vi "Actor Core.vi"(8 "error in":errorcluster, 11 "SongPlayerActor in":refnum<class "SongPlayerActor.lvclass">) -> (0 "error out":errorcluster, 3 "Actor out":refnum<class "Actor.lvclass">)   [LabVIEW 2015, in "SongPlayerActor.lvlib" / "SongPlayerActor.lvclass"]
doc: "(<B>Filename</B>: Actor Framework.lvlib:Actor.lvclass:Actor Core.vi)\n\nReceives messages to the actor, reacts to them, and initiates any error handling that may shut the actor down.\n\nDescendant classes may override this VI to append parallel tasks for the actor to complete while it handles messages. Overrides use the Call Parent Method node."
uses:
  SongPlayerActor.lvclass
  <vilib>/ActorFramework/Actor/Actor.lvclass
  file/MusicElement/Song/Song Duration.ctl
  file/MusicElement/Song/Song.lvclass
  SongPlayerActor.lvclass/SongPlayerActor.ctl
  <vilib>/ActorFramework/Actor/Actor.lvclass/Actor.ctl
  <vilib>/ActorFramework/Message Enqueuer/Message Enqueuer.lvclass/Message Enqueuer.ctl
  file/MusicElement/Song/Song.lvclass/Song.ctl
  file/MusicElement/MusicElement.lvclass/MusicElement.ctl
  file/MusicElement/Read Name.vi
  file/MusicElement/Song/Read Artist.vi
  file/MusicElement/Song/Read Album.vi
  <vilib>/ActorFramework/Message Enqueuer/Init from Existing Queue.vi
  <vilib>/ActorFramework/Message Enqueuer/Enqueue.vi
  <vilib>/ActorFramework/Message Priority Queue/Priority Enqueue.vi
  <vilib>/ActorFramework/Message Enqueuer/Message Enqueuer.lvclass
  <vilib>/ActorFramework/Stop Msg/Stop Msg.lvclass
  SongQueueActor/SongQueueActor Messages/Dequeue Next Song Msg/Dequeue Next Song Msg.lvclass
  SongQueueActor/SongQueueActor Messages/Play Previous Song Msg/Play Previous Song Msg.lvclass
panel:
  out "Main UI":enum32{"Main", "Debug"}(tab)
  out "Time Remaining (s)":T1 format="%<%M:%S>T"
  in  "Song Progress (%)":dbl(slide) scale=0.0..1.0
  in  "Paused?":bool
  in  "Previous Song":bool
  in  "Next Song":bool
  out "Artist":string
  out "Album":string
  out "Song Name":string
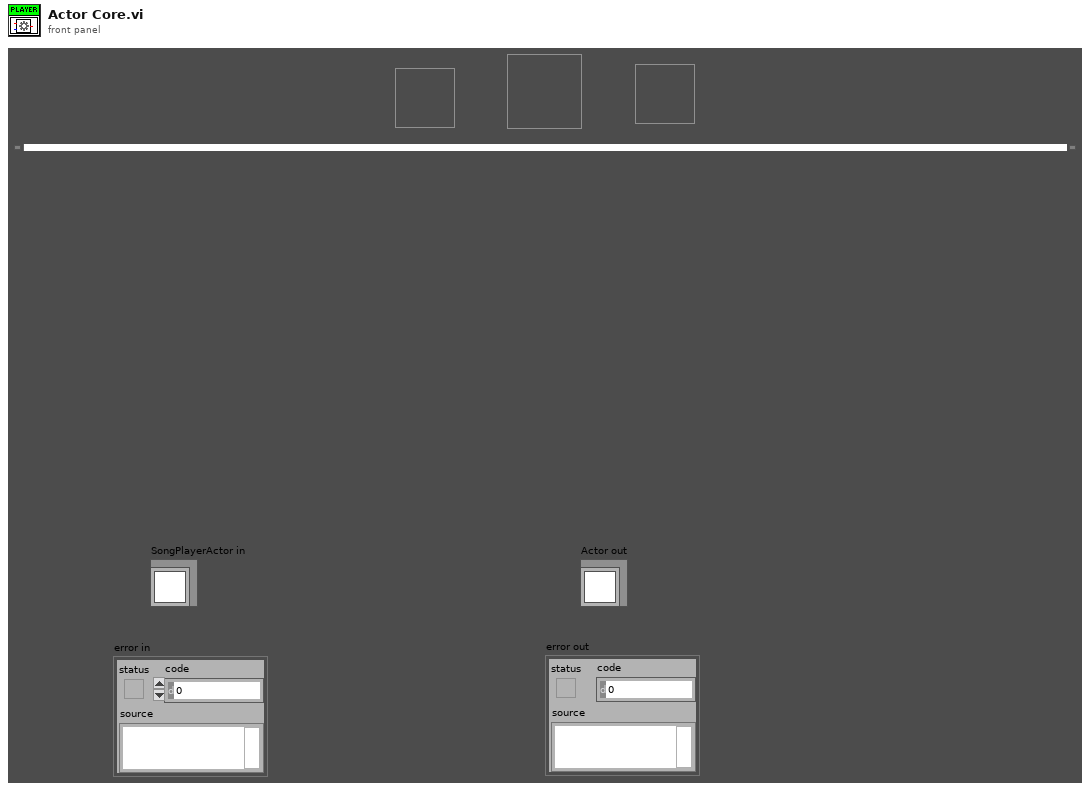
[diagram p1: front panel]
types:
  T1 = typedef "Song.lvclass/Song Duration.ctl" = timestamp
  T2 = enum8{"Enabled", "Disabled", "Disabled and Grayed Out"}
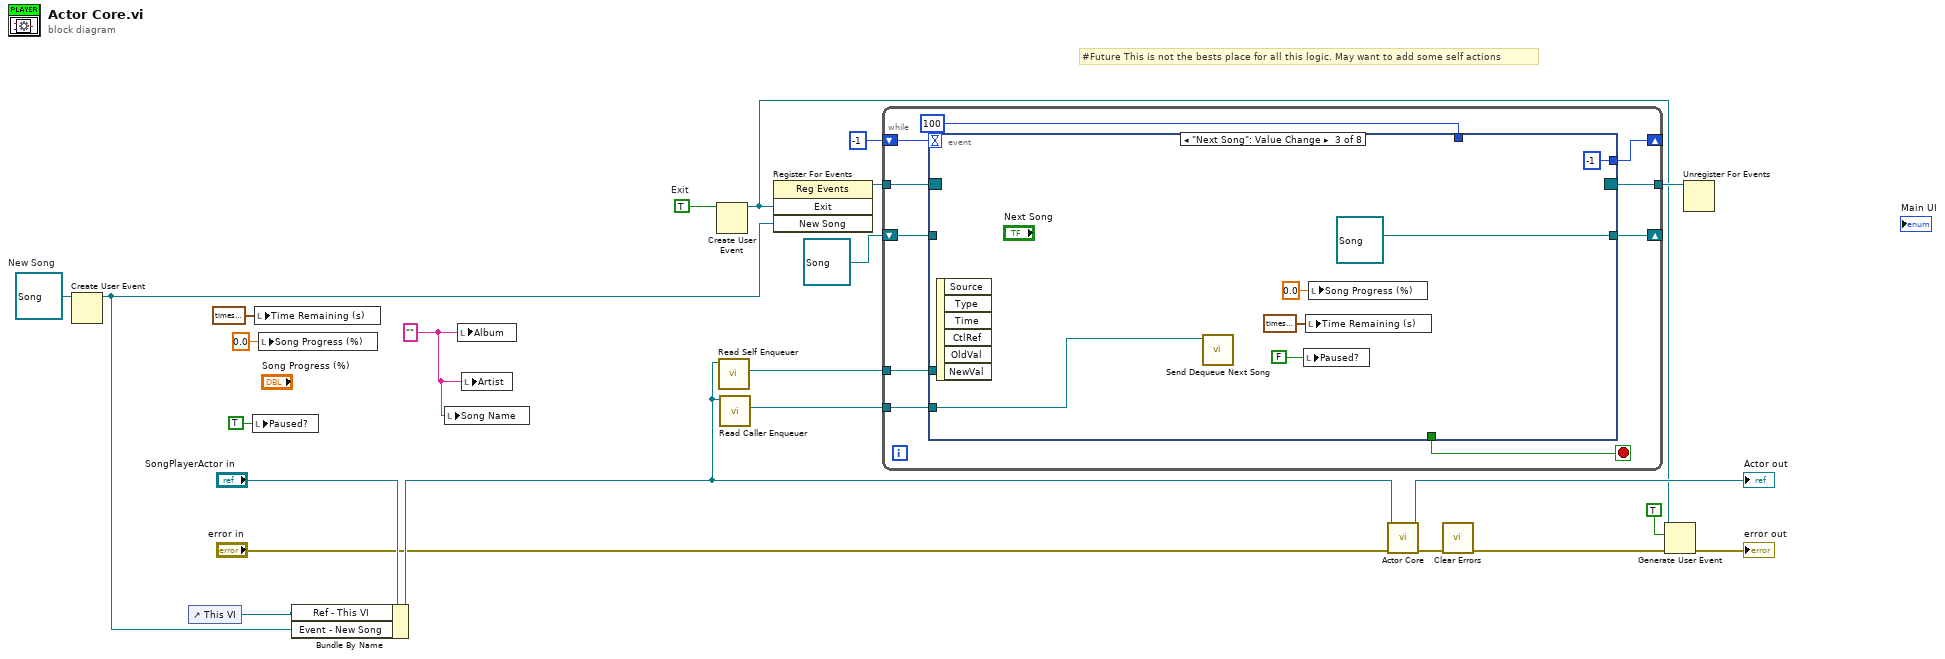
[diagram p0: block diagram]
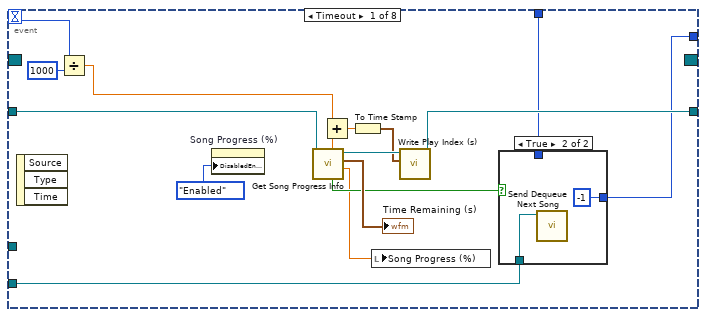
[diagram p2: hidden frame]
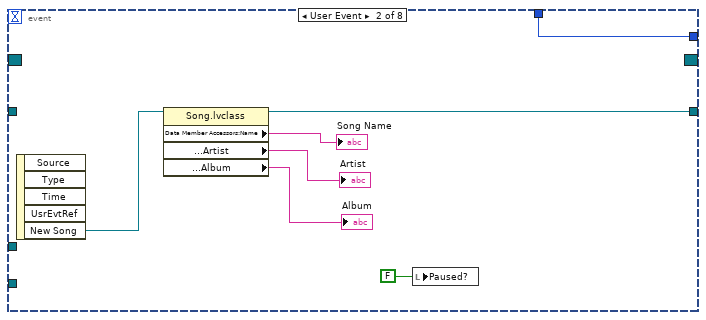
[diagram p4: hidden frame]
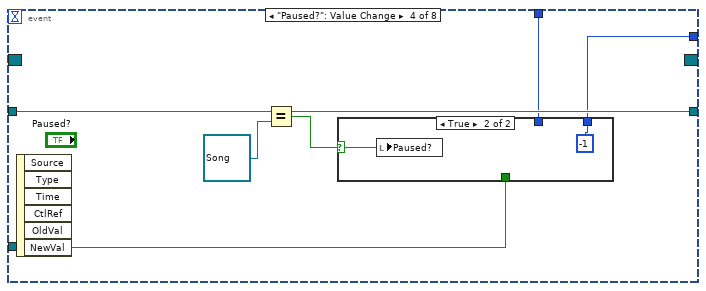
[diagram p5: hidden frame]
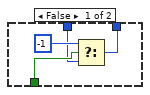
[diagram p6: hidden frame]
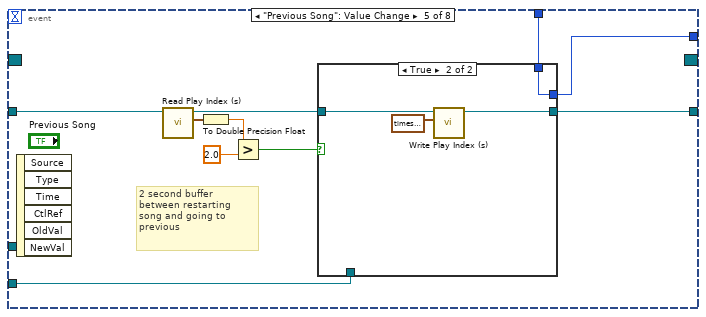
[diagram p7: hidden frame]
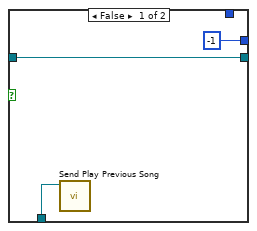
[diagram p8: hidden frame]
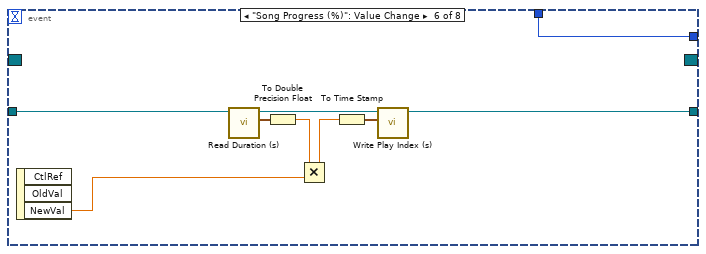
[diagram p9: hidden frame]
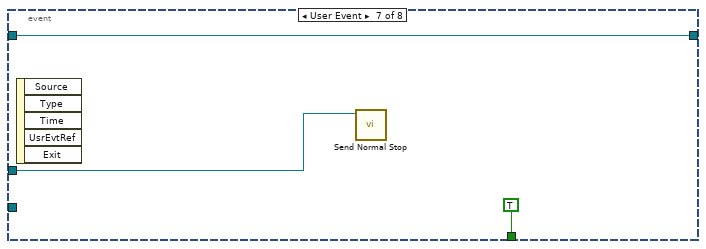
[diagram p10: hidden frame]
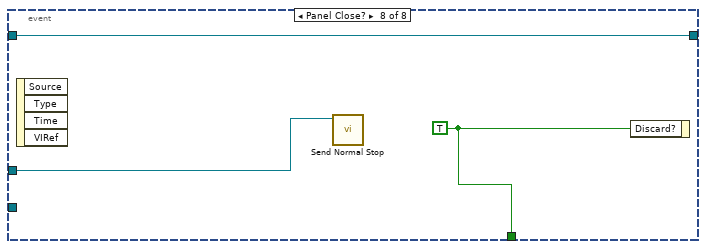
[diagram p11: hidden frame]
diagram:
  w2 = "" ("Album")
  w13 = refnum<class "Song.lvclass"> refnum  # New Song
  w22 = TRUE  # Exit
  # "#Future This is not the bests place for all this logic. May want to add some self actions"
  n1 = Create User Event(user event datatype=w13) -> (user event=w6:refnum<user-event>)  [unwired: 1 in, 1 out]
  n2 = control-ref of="This VI"() -> (w7:refnum<vi>)
  n3 = local write "Paused?"(TRUE ("Paused?")) -> ()
  n4 = local write "Time Remaining (s)"(T1 timestamp(0 s since 1904-01-01) ("Time Remaining (s)")) -> ()
  n5 = local write "Song Progress (%)"(0.0 ("Song Progress (%)")) -> ()
  n6 = Bundle By Name(cluster="SongPlayerActor in", "Ref - This VI"=w7, "Event - New Song"=w6) -> (w8:refnum<class "SongPlayerActor.lvclass">)
  n7 = local write "Song Name"(w2) -> ()
  n8 = local write "Album"(w2) -> ()
  n9 = local write "Artist"(w2) -> ()
  n10 = Create User Event(user event datatype=w22) -> (user event=w14:refnum<user-event>)  [unwired: 1 in, 1 out]
  n11 = call <vilib>:"Read Self Enqueuer.vi"("Actor"=w8) -> ("Self Enqueuer"=w15:refnum<class "Message Enqueuer.lvclass">)  [unwired: 10 in]
  n12 = call <vilib>:"Read Caller Enqueuer.vi"("Actor"=w8) -> ("Caller Enqueuer"=w12:refnum<class "Message Enqueuer.lvclass">)  [unwired: 10 in]
  n13 = register-events(w14, w6) -> (reference out=w21:refnum<event-registration>)  [unwired: 2 in, 1 out]
  n14 = while {
    tunnel: w21 -> [w33]
    tunnel: [w31] -> w20
    tunnel: w15 -> [w30]
    shift-right: [w29] -> _
    shift-left: refnum<class "Song.lvclass"> refnum ("Song out") -> [w28]
    tunnel: w12 -> [w27]
    shift-right: [w25] -> _
    shift-left: -1 -> [w26]
    stop <- w32 stop-if-true
    n15 = event shown="[2] \"Next Song\": Value Change" {
      selector: w33 -> [_ _ _ _ _ _ _ _]
      dyn-events: [_ _ _ _ _ _ _ _] -> w31
      timeout: w26 -> [w44 _ _ _ _ _ _ _]
      tunnel: [_ _ _ _ _ _ TRUE ("Exit") w109] -> w32
      tunnel: w30 -> [_ _ _ _ _ _ w105 w108]
      tunnel: [w49 w57 refnum<class "Song.lvclass"> refnum ("New Song") w69 w81 w99 w104 w107] -> w29
      tunnel: w28 -> [w45 _ _ w69 w87 w102 w104 w107]
      tunnel: w27 -> [w46 _ w65 _ w80 _ _ _]
      tunnel: [w43 w53 -1 w66 w79 w95 _ _] -> w25
      tunnel: 100 -> [w42 w53 _ w67 w78 w95 _ _]
      event Timeout {
        n16 = event-data() -> ()  [unwired: 1 in, 3 out]
        n17 = Divide(x=w44, y=1000) -> (x/y=w47:dbl)
        n18 = property on="Song Progress (%)" class="Slide (strict)"("DisabledEnum"=T2."Enabled" ("Disabled")) -> ()  [unwired: 2 in, 2 out]
        n19 = call "Get Song Progress Info.vi"("Song in"=w45) -> ("Percent Complete"=w34:dbl, "Time Remaining (s)"=→"Time Remaining (s)":T1, "Song out"=w40:refnum<class "Song.lvclass">, "Complete?"=w35:bool, "Time Complete (s)"=w39:dbl)  [unwired: 5 in, 1 out]
        n20 = Add(x=w47, y=w39) -> (x+y=w38:dbl)
        n21 = To Time Stamp(1:w38) -> (0:w37:timestamp)
        n22 = local write "Song Progress (%)"(w34) -> ()
        n23 = call "Write Play Index (s).vi"("Play Index (s)"=w37, "Song in"=w40) -> ("Song out"=w49:refnum<class "Song.lvclass">)  [unwired: 8 in, 1 out]
        n24 = case shown="True" w35 {
          tunnel: w46 -> [_ w52]
          tunnel: [w50 -1] -> w43
          tunnel: w42 -> [w50 _]
          frame False {
          }
          frame True {
            n25 = call "Send Dequeue Next Song.vi"("Message Enqueuer in"=w52) -> ()  [unwired: 9 in, 2 out]
          }
        }
      }
      event User Event {
        n26 = event-data() -> ("New Song"=w58:refnum<class "Song.lvclass">)  [unwired: 1 in, 4 out]
        n27 = property class="Song.lvclass"(reference=w58) -> (reference out=w57:refnum<class "Song.lvclass">, "Data Member Accessors:Name"=→"Song Name":string, "API:Data Member Accessors:Artist"=→"Artist":string, "API:Data Member Accessors:Album"=→"Album":string)  [unwired: 1 in, 1 out]
        n28 = local write "Paused?"(FALSE ("Play/Pause")) -> ()
      }
      event "Next Song": Value Change {
        n29 = event-data() -> ()  [unwired: 1 in, 6 out]
        n30 = call "Send Dequeue Next Song.vi"("Message Enqueuer in"=w65) -> ()  [unwired: 9 in, 2 out]
        n31 = local write "Paused?"(FALSE ("Play/Pause")) -> ()
        n32 = local write "Time Remaining (s)"(T1 timestamp(0 s since 1904-01-01) ("Time Remaining (s)")) -> ()
        n33 = local write "Song Progress (%)"(0.0 ("Song Progress (%)")) -> ()
      }
      event "Paused?": Value Change {
        n34 = event-data() -> ("NewVal"=w68:bool)  [unwired: 1 in, 5 out]
        n35 = Equal?(x=w69, y=refnum<class "Song.lvclass"> refnum ("Song out")) -> (x = y?=w70:bool)
        n36 = case shown="True" w70 {
          selector: w70 -> [_ w77]
          tunnel: w68 -> [w75 _]
          tunnel: w67 -> [w73 _]
          tunnel: [w72 -1] -> w66
          frame False {
            n37 = Select(t=-1, s=w75, f=w73) -> (s? t:f=w72:i32)
          }
          frame True {
            n38 = local write "Paused?"(w77) -> ()
          }
        }
      }
      event "Previous Song": Value Change {
        # "2 second buffer between restarting song and going to previous"
        n39 = event-data() -> ()  [unwired: 1 in, 6 out]
        n40 = call "Read Play Index (s).vi"("Song in"=w87) -> ("Play Index (s)"=w86:T1, "Song out"=w82:refnum<class "Song.lvclass">)  [unwired: 8 in, 1 out]
        n41 = To Double Precision Float(number=w86) -> (double precision float=w85:dbl)
        n42 = Greater?(x=w85, y=2.0 ("double precision float")) -> (0:w83:bool)
        n43 = case shown="True" w83 {
          tunnel: w82 -> [w90 w94]
          tunnel: [w90 w92] -> w81
          tunnel: w80 -> [w89 _]
          tunnel: [-1 w91] -> w79
          tunnel: w78 -> [_ w91]
          frame False {
            n44 = call "Send Play Previous Song.vi"("Message Enqueuer in"=w89) -> ()  [unwired: 9 in, 2 out]
          }
          frame True {
            n45 = call "Write Play Index (s).vi"("Play Index (s)"=T1 timestamp(0 s since 1904-01-01), "Song in"=w94) -> ("Song out"=w92:refnum<class "Song.lvclass">)  [unwired: 8 in, 1 out]
          }
        }
      }
      event "Song Progress (%)": Value Change {
        n46 = event-data() -> ("NewVal"=w103:dbl)  [unwired: 1 in, 2 out]
        n47 = call "Read Duration (s).vi"("Song in"=w102) -> ("Duration (s)"=w101:T1, "Song out"=w100:refnum<class "Song.lvclass">)  [unwired: 8 in, 1 out]
        n48 = To Double Precision Float(number=w101) -> (double precision float=w97:dbl)
        n49 = Multiply(x=w97, y=w103) -> (x*y=w96:dbl)
        n50 = To Time Stamp(1:w96) -> (0:w98:timestamp)
        n51 = call "Write Play Index (s).vi"("Play Index (s)"=w98, "Song in"=w100) -> ("Song out"=w99:refnum<class "Song.lvclass">)  [unwired: 8 in, 1 out]
      }
      event User Event {
        n52 = event-data() -> ()  [unwired: 1 in, 5 out]
        n53 = call <vilib>:"Send Normal Stop.vi"("Message Enqueuer"=w105) -> ()  [unwired: 10 in, 1 out]
      }
      event Panel Close? {
        w109 = TRUE ("Discard?")
        n54 = event-data() -> ()  [unwired: 1 in, 4 out]
        n55 = call <vilib>:"Send Normal Stop.vi"("Message Enqueuer"=w108) -> ()  [unwired: 10 in, 1 out]
        n56 = event-data("Discard?"=w109) -> ()  [unwired: 1 in, 1 out]
      }
    }
  }
  n57 = call-parent "Actor Core.vi"("error in"="error in", "Actor in"=w8) -> ("error out"=w19:errorcluster, "Actor out"=→"Actor out":refnum<class "Actor.lvclass">)  [unwired: 8 in]
  n58 = call <vilib>:"Clear Errors.vi"("error in (no error)"=w19) -> ("error out"=w17:errorcluster)  [unwired: 5 in, 1 out]
  n59 = Generate User Event(user event=w14, event data cluster=TRUE ("event data"), error in=w17) -> (error out=→"error out":errorcluster)  [unwired: 1 in, 1 out]
  n60 = Unregister For Events(event registration refnum=w20) -> ()  [unwired: 1 in, 1 out]
